vi "Rotate24bitGaugePixmap.vi"(7 "Maske kombinieren? (F)":bool, 9 "Rotation Angle (degrees)":dbl format="%.2f", 10 "Größe des Darstellungsbereichs":T2, 11 "image data":T1 caption="Bilddaten") -> (3 "image data out":T1 caption="Bilddaten")   [LabVIEW 2017]
doc: "Used for 24 bit pixmaps."
uses:
  <vilib>/Utility/miscctls.llb/LVBoundsTypeDef.ctl
  <vilib>/picture/picture.llb/imagedata.ctl
panel:
  out "GaugePicture":picture
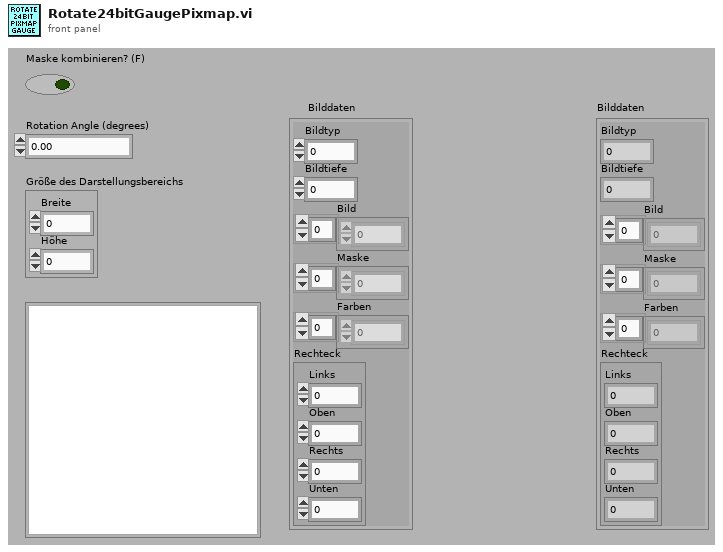
[diagram p1: front panel]
types:
  T1 = typedef "imagedata.ctl" = cluster{"image type":i32, "image depth":i32, "image":u8[], "mask":u8[], "colors":u32[], "Rectangle":cluster{"left":i16, "top":i16, "right":i16, "bottom":i16}}
  T2 = typedef "LVBoundsTypeDef.ctl" = cluster{"Width":u32, "Height":u32}
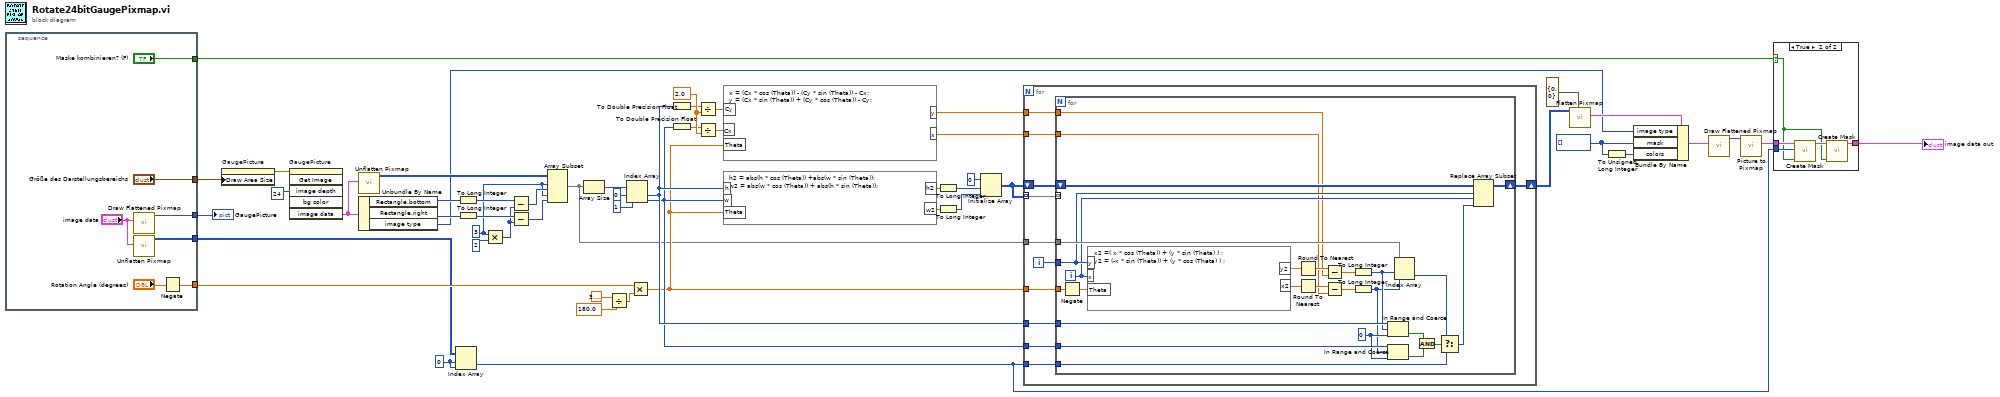
[diagram p0: block diagram]
diagram:
  w8 = 0 ("index (row)")
  w13 = u8[] [] ("mask")
  w18 = 3 ("Array Index")
  w38 = 2.0 ("y")
  n1 = stacked-sequence {
    tunnel: [w58] -> w53
    tunnel: ["Größe des Darstellungsbereichs"] -> w30
    tunnel: [w57] -> w9
    tunnel: [w55] -> w3
    tunnel: ["Maske kombinieren? (F)"] -> w1
    frame #0 {
      n2 = call <vilib>:"Draw Flattened Pixmap.vi"("image data"="image data") -> ("new picture"=w57:picture)  [unwired: 1 in, 7 out]
      n3 = call <vilib>:"Unflatten Pixmap.vi"("image data"="image data") -> ("24-bit pixmap"=w55:u32[][])  [unwired: 4 in, 6 out]
      n4 = Negate(x="Rotation Angle (degrees)") -> (-x=w58:dbl)
    }
  }
  "GaugePicture" <- w9
  n5 = property on="GaugePicture" class="Pict"("Draw Area Size"=w30) -> (error out=w29:errorcluster)  [unwired: 2 in, 1 out]
  n6 = invoke on="GaugePicture" class="Bild" method="Get Image"(error in=w29, "image depth"=24 ("Bildtiefe")) -> ("image data"=w27:T1)  [unwired: 4 in, 5 out]
  n7 = call <vilib>:"Unflatten Pixmap.vi"("image data"=w27) -> ("24-bit pixmap"=w7:u32[][])  [unwired: 4 in, 6 out]
  n8 = Unbundle By Name(w27) -> ("Rectangle.bottom"=w26:i16, "Rectangle.right"=w24:i16, "image type"=w4:i32)
  n9 = Index Array(array=w3, index (row)=w8, index (col)=w8) -> (element=w2:u32)
  n10 = To Long Integer(number=w26) -> (32bit integer=w25:i32)
  n11 = To Long Integer(number=w24) -> (32bit integer=w23:i32)
  n12 = Multiply(x=w18, y=2) -> (x*y=w19:i32)
  n13 = Subtract(x=w25, y=w19) -> (x-y=w22:i32)
  n14 = Subtract(x=w23, y=w19) -> (x-y=w21:i32)
  n15 = Array Subset(array=w7, index (row)=w18, length (row)=w22, index (col)=w18, length (col)=w21) -> (w17:u32[][])
  n16 = Array Size(array=w17) -> (size(s)=w47:i32[])
  n17 = Divide(x=3.141592653589793, y=180.0) -> (x/y=w52:dbl)
  n18 = Index Array(array=w47, index #1=0 ("Index"), index #2=1 ("Index")) -> (element #1=w35:i32, element #2=w34:i32)
  n19 = Multiply(x=w53, y=w52) -> (x*y=w33:dbl)
  n20 = To Double Precision Float(number=w35) -> (double precision float=w37:dbl)
  n21 = To Double Precision Float(number=w34) -> (double precision float=w36:dbl)
  n22 = Divide(x=w37, y=w38) -> (x/y=w39:dbl)
  n23 = Divide(x=w36, y=w38) -> (x/y=w40:dbl)
  n24 = formula code="x = (Cx * cos (Theta)) - (Cy * sin (Theta)) - Cx;\ny = (Cx * sin (Theta)) + (Cy * cos (Theta)) - Cy;"("Cx"=w40, "Cy"=w39, "Theta"=w33) -> ("x"=w32:dbl, "y"=w31:dbl)
  n25 = formula code="h2 = abs(h * cos (Theta)) +abs(w * sin (Theta)); \nw2 = abs(w * cos (Theta)) + abs(h * sin (Theta));"("h"=w35, "w"=w34, "Theta"=w33) -> ("h2"=w43:dbl, "w2"=w44:dbl)
  n26 = To Long Integer(number=w43) -> (32bit integer=w42:i32)
  n27 = To Long Integer(number=w44) -> (32bit integer=w41:i32)
  n28 = Initialize Array(u32 0, w42, w41) -> (w45:u32[][])
  n29 = for {
    tunnel: w17 -> [w71]
    tunnel: w33 -> [w66]
    shift-right: [w69] -> w15
    shift-left: w45 -> [w68]
    tunnel: w45 -> [w67] mode=indexing
    tunnel: w34 -> [w65]
    tunnel: w35 -> [w64]
    tunnel: w32 -> [w63]
    tunnel: w31 -> [w62]
    tunnel: w2 -> [w61]
    i -> [w70]
    n30 = for {
      tunnel: w71 -> [w92]
      tunnel: w70 -> [w90]
      tunnel: w66 -> [w93]
      shift-right: [w95] -> w69
      shift-left: w68 -> [w94]
      tunnel: w67 -> [_] mode=indexing
      tunnel: w65 -> [w85]
      tunnel: w64 -> [w86]
      tunnel: w63 -> [w77]
      tunnel: w62 -> [w76]
      tunnel: w61 -> [w74]
      i -> [w89]
      w75 = 0 ("lower limit")
      n31 = Negate(x=w93) -> (-x=w91:dbl)
      n32 = formula code="x2 =( x * cos (Theta)) + (y * sin (Theta) ) ;\ny2 = (-x * sin (Theta)) + (y * cos (Theta) ) ;"("y"=w90, "x"=w89, "Theta"=w91) -> ("y2"=w97:dbl, "x2"=w96:dbl)
      n33 = Round To Nearest(number=w97) -> (nearest integer value=w88:dbl)
      n34 = Round To Nearest(number=w96) -> (nearest integer value=w87:dbl)
      n35 = Subtract(x=w88, y=w76) -> (x-y=w83:dbl)
      n36 = Subtract(x=w87, y=w77) -> (x-y=w84:dbl)
      n37 = To Long Integer(number=w83) -> (32bit integer=w73:i32)
      n38 = To Long Integer(number=w84) -> (32bit integer=w72:i32)
      n39 = In Range and Coerce(upper limit=w86, x=w73, lower limit=w75) -> (In Range?=w81:bool)  [unwired: 1 out]
      n40 = In Range and Coerce(upper limit=w85, x=w72, lower limit=w75) -> (In Range?=w80:bool)  [unwired: 1 out]
      n41 = Index Array(array=w92, index (row)=w73, index (col)=w72) -> (element=w82:u32)
      n42 = And(x=w81, y=w80) -> (x .and. y?=w79:bool)
      n43 = Select(t=w82, s=w79, f=w74) -> (s? t:f=w78:u32)
      n44 = Replace Array Subset(array=w94, new element=w78, index (row)=w90, index (col)=w89) -> (w95:u32[][])
    }
  }
  n45 = call <vilib>:"Flatten Pixmap.vi"("top left"=cluster{"x":i16, "y":i16} {"x"=0, "y"=0}, "24-bit pixmap"=w15) -> ("image data"=w14:T1)  [unwired: 9 in]
  n46 = To Unsigned Long Integer(number=w13) -> (unsigned 32bit integer=w12:u32[])
  n47 = Bundle By Name(cluster=w14, "image type"=w4, "mask"=w13, "colors"=w12) -> (w11:T1)
  n48 = call <vilib>:"Draw Flattened Pixmap.vi"("image data"=w11) -> ("new picture"=w10:picture)  [unwired: 8 in]
  n49 = call <vilib>:"Picture to Pixmap.vi"("picture"=w10) -> ("image data"=w6:T1)  [unwired: 3 in, 7 out]
  n50 = case shown="True" w1 {
    selector: w1 -> [_ w99]
    tunnel: w6 -> [w98 w103]
    tunnel: [w98 w101] -> w5
    tunnel: w2 -> [_ w100]
    frame False {
    }
    frame True {
      n51 = call <vilib>:"Create Mask.vi"("Combine Masks? (F)"=w99, "Mask Color (Black)"=w100, "image data"=w103) -> ("image data"=w102:T1)  [unwired: 1 in, 7 out]
      n52 = call <vilib>:"Create Mask.vi"("Combine Masks? (F)"=w99, "image data"=w102) -> ("image data"=w101:T1)  [unwired: 2 in, 7 out]
    }
  }
  "image data out" <- w5
